vi "Get Session Information.vi"(8 "error in (no error)":errorcluster, 11 "session information":T1[](array[typedef])) -> (0 "error out":errorcluster, 3 "session information":T1)   [LabVIEW 2021, in "Measurement Service Helpers.lvlib"]
doc: "Returns the first session information based on the given list of session information."
uses:
  Measurement Service Helpers.lvlib
  <vilib>/MeasurementLink/MeasurementLink Session Management Client/RPC Messages/ni_measurementlink_sessionmanagement_v1_SessionInformation.ctl
  <vilib>/MeasurementLink/MeasurementLink Session Management Client/RPC Messages/nidevice_grpc_Session.ctl
  <vilib>/MeasurementLink/MeasurementLink Session Management Client/RPC Messages/ni_measurementlink_sessionmanagement_v1_ChannelMapping.ctl
  <vilib>/MeasurementLink/MeasurementLink Session Management Client/MeasurementLink Session Management Client.lvlib
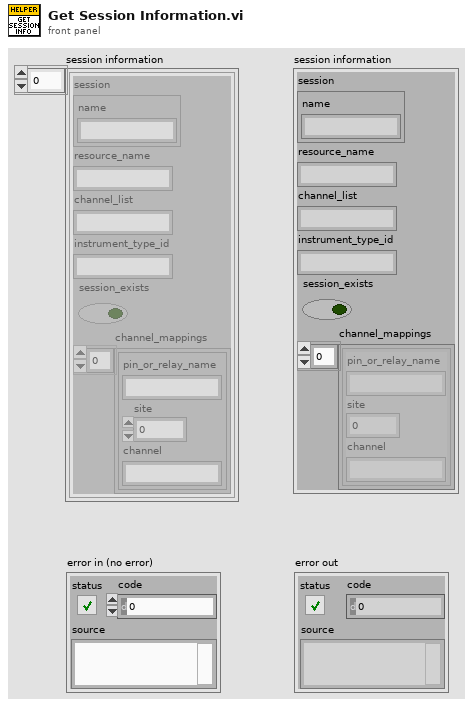
[diagram p1: front panel]
types:
  T1 = typedef "MeasurementLink Session Management Client.lvlib/ni_measurementlink_sessionmanagement_v1_SessionInformation.ctl" = cluster{"session":T2, "resource_name":string, "channel_list":string, "instrument_type_id":string, "session_exists":bool, "channel_mappings":T3[]}
  T2 = typedef "MeasurementLink Session Management Client.lvlib/nidevice_grpc_Session.ctl" = cluster{"name":string}
  T3 = typedef "MeasurementLink Session Management Client.lvlib/ni_measurementlink_sessionmanagement_v1_ChannelMapping.ctl" = cluster{"pin_or_relay_name":string, "site":i32, "channel":string}
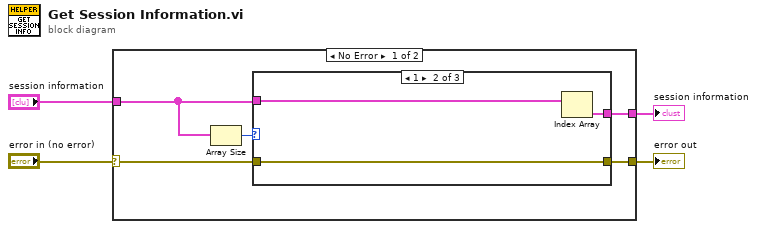
[diagram p0: block diagram]
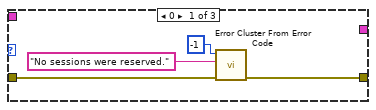
[diagram p2: hidden frame]
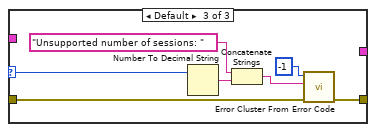
[diagram p3: hidden frame]
diagram:
  n1 = case shown="No Error" "error in (no error)" {
    selector: "error in (no error)" -> [w8 w24]
    tunnel: "session information" -> [w5 _]
    tunnel: [w7 w24] -> w3
    tunnel: [w6 _] -> w1
    frame No Error {
      n2 = Array Size(array=w5) -> (size(s)=w9:i32)
      n3 = case shown="1" w9 {
        selector: w9 -> [_ _ w18]
        tunnel: w8 -> [w13 w15 w23]
        tunnel: [w10 w15 w21] -> w7
        tunnel: w5 -> [_ w14 _]
        tunnel: [_ w16 _] -> w6
        frame 0 {
          n4 = call <vilib>:"Error Cluster From Error Code.vi"("error in (no error)"=w13, "error message (\"\")"="No sessions were reserved." ("error message (\"\")"), "error code (0)"=-1) -> ("error out"=w10:errorcluster)  [unwired: 6 in]
        }
        frame 1 {
          n5 = Index Array(array=w14) -> (element=w16:T1)  [unwired: 1 in]
        }
        frame Default {
          n6 = Number To Decimal String(number=w18) -> (decimal integer string=w19:string)  [unwired: 1 in]
          n7 = Concatenate Strings("Unsupported number of sessions: " ("error message (\"\")"), w19) -> (w17:string)
          n8 = call <vilib>:"Error Cluster From Error Code.vi"("error in (no error)"=w23, "error message (\"\")"=w17, "error code (0)"=-1) -> ("error out"=w21:errorcluster)  [unwired: 6 in]
        }
      }
    }
    frame Error {
    }
  }
  "error out" <- w3
  "session information" <- w1
